vi "NIIE_Prepare Glyphs for Display.vi"(1 "Icon Templates":T2[](array[typedef])) -> (0 "Array Out":T1[][](array[typedef]))   [LabVIEW 2021]
uses:
  MB CORE/TypeDefs/Cluster_Path&Icon.ctl
  vi.lib/LabVIEW Icon API/lv_icon/Controls/Graphic.ctl
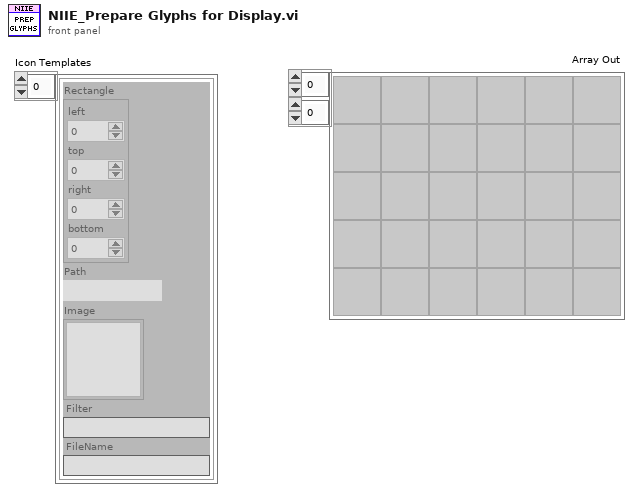
[diagram p1: front panel]
types:
  T1 = typedef "Graphic.ctl" = cluster{"Rectangle":cluster{"left":i16, "top":i16, "right":i16, "bottom":i16}, "Path":path, "Image":picture, "Filter":string, "FileName":string}
  T2 = typedef "Cluster_Path&Icon.ctl" = cluster{"Rectangle":cluster{"left":i16, "top":i16, "right":i16, "bottom":i16}, "Path":path, "Image":picture, "Filter":string, "FileName":string}
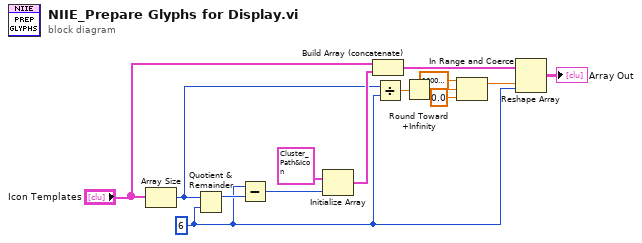
[diagram p0: block diagram]
diagram:
  w1 = 6 ("y")
  n1 = Array Size(array="Icon Templates") -> (size(s)=w7:i32)
  n2 = Quotient & Remainder(x=w7, y=w1) -> (x-y*floor(x/y)=w5:i32)  [unwired: 1 out]
  n3 = Subtract(x=w1, y=w5) -> (x-y=w6:i32)
  n4 = Initialize Array(T2 {"Rectangle"={"left"=0, "top"=0, "right"=0, "bottom"=0}, "Path"=path "", "Image"=bytes[0], "Filter"="", "FileName"=""} ("Path & Icon"), w6) -> (w12:T2[])
  n5 = Build Array (concatenate)("Icon Templates", w12) -> (w4:T2[])
  n6 = Divide(x=w7, y=w1) -> (x/y=w3:dbl)
  n7 = Round Toward +Infinity(x=w3) -> (ceil(x): smallest int >= x=w8:dbl)
  n8 = In Range and Coerce(upper limit=10000000.0, x=w8, lower limit=0.0) -> (coerced(x)=w11:dbl)  [unwired: 1 out]
  n9 = Reshape Array(w4, w11, w1) -> (→"Array Out":T2[][])
